vi "vision info 2.vi"() -> ()   [LabVIEW 2018]
uses:
  <vilib>/userdefined/High Color/IMAQdx.ctl
panel:
  out "Session Out":T1
  out "Type line 2":enum16{"Z", "I", "O", "S", "L", "J", "T", "N"}(ring)
  out "Type line 1":enum16{"Z", "I", "O", "S", "L", "J", "T", "N"}(ring)
  out "Type region 3":enum16{"Z", "I", "O", "S", "L", "J", "T", "N"}(ring)
  out "Type region 2":enum16{"Z", "I", "O", "S", "L", "J", "T", "N"}(ring)
  out "Type region 1":enum16{"Z", "I", "O", "S", "L", "J", "T", "N"}(ring)
  in  "c4":i8
  in  "c3":i8
  in  "stop vision cube":bool
  out "cube detected":bool
  in  "c2":i8
  in  "c1":i8
  out "_y":dbl
  out "_x":dbl
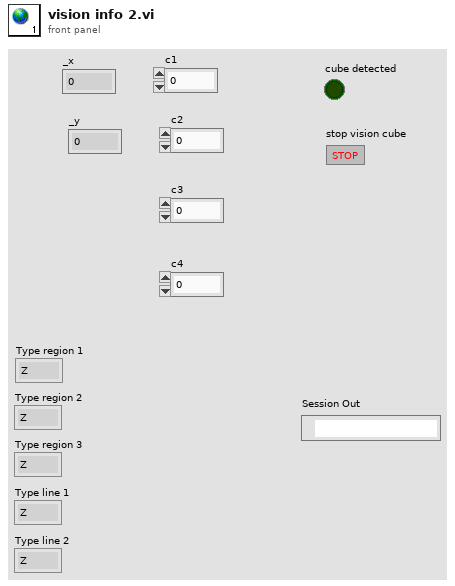
[diagram p1: front panel]
types:
  T1 = typedef "IMAQdx.ctl" = refnum<k21>
diagram:
